vi "Page_Version_Initialize.vi"(6 "output cluster":T1, 8 "error in (no error)":errorcluster, 11 "AB_Build in":refnum<class "AB_Build.lvclass">) -> (0 "error out":errorcluster, 3 "AB_Build out":refnum<class "AB_Build.lvclass">)   [LabVIEW 2020, in "AB_Build.lvclass"]
uses:
  <vilib>/AppBuilder/AB_Classes/Build/AB_Build.lvclass
  <resource>/Framework/Providers/Builds/AppBuilder/AB_UI_Page_Version_References.ctl
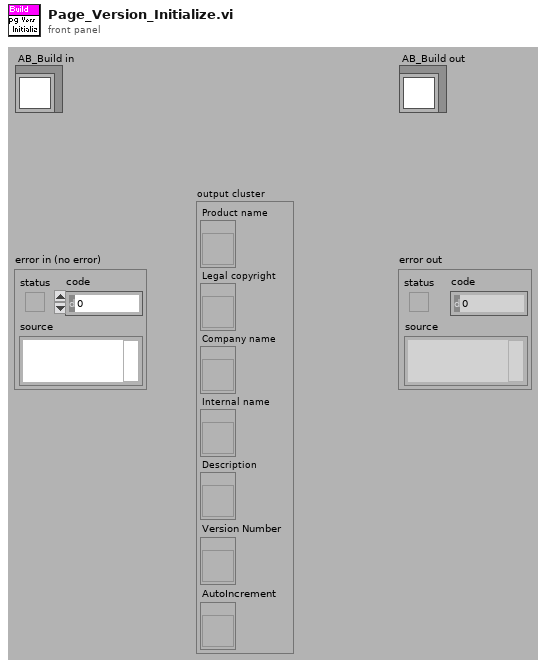
[diagram p1: front panel]
types:
  T1 = typedef "AB_UI_Page_Version_References.ctl" = cluster{"Product name":refnum<vi>, "Legal copyright":refnum<vi>, "Company name":refnum<vi>, "Internal name":refnum<vi>, "Description":refnum<vi>, "Version Number":refnum<vi>, "AutoIncrement":refnum<vi>}
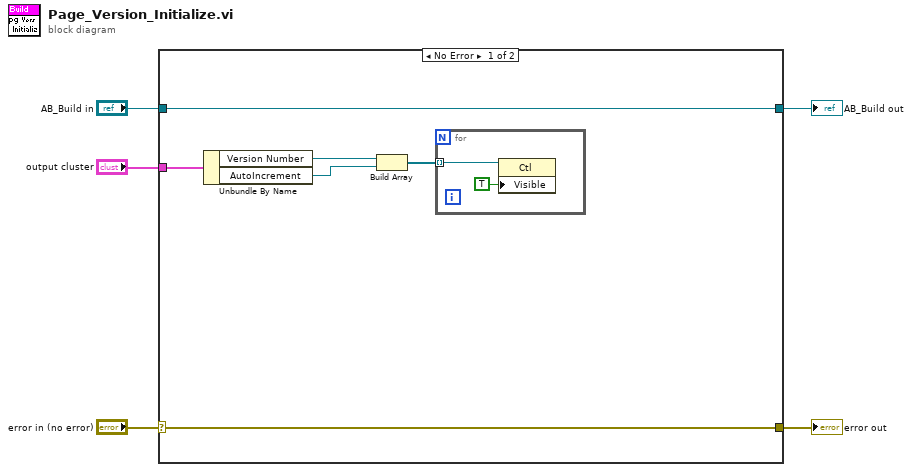
[diagram p0: block diagram]
diagram:
  n1 = case shown="No Error" "error in (no error)" {
    selector: "error in (no error)" -> [w10 w15]
    tunnel: [w10 w15] -> w2
    tunnel: [w11 w14] -> w4
    tunnel: "AB_Build in" -> [w11 w14]
    tunnel: "output cluster" -> [w9 _]
    frame No Error {
      n2 = Unbundle By Name(w9) -> ("Version Number"=w8:refnum<vi>, "AutoIncrement"=w7:refnum<vi>)
      n3 = Build Array(w8, w7) -> (w6:refnum<vi>[])
      n4 = for {
        tunnel: w6 -> [w13] mode=indexing
        n5 = property class="Ctl"(reference=w13, "Visible"=TRUE) -> ()  [unwired: 1 in, 2 out]
      }
    }
    frame Error {
    }
  }
  "error out" <- w2
  "AB_Build out" <- w4
